vi "GlobalClicksHeight_flt.vi"() -> ()   [LabVIEW 2017]
panel:
  in  "Starting Height?":bool
  in  "Clicks and Height":bool
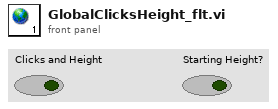
[diagram p1: front panel]
diagram:
